vi "InitFpga.vi"(6 "bitfile path":path, 8 "error in (no error)":errorcluster, 10 "Device Name":refnum<k15>="RIO0", 11 "FPGA ref":T1) -> (0 "error out":errorcluster, 2 "session handle out":refnum<k15>, 3 "FPGA ref out":T1)   [LabVIEW 2025]
uses:
  <vilib>/rvi/interface/nirviReadWriteControl/nirviReadWriteControl.xnode
  NiFpgaLv.dll
  <vilib>/Utility/error.llb/Error Cluster From Error Code.vi
  <vilib>/rvi/interface/Simulation/niFpgaSimulationCallBeginRW.vi
  <vilib>/rvi/errors/niLvFpgaAdjustHostInterfaceError.vi
  <vilib>/rvi/interface/nirviMethod/nirviMethod.xnode
  <vilib>/rvi/errors/niLvFpgaMergeErrorWithErrorCode.vi
  x410-fpga-ref.ctl
  <vilib>/FPGAPlugInAG/Dynamic/niLvFpga_ConfigureFifo_Dynamic.vi
  <vilib>/FPGAPlugInAG/Dynamic/niLvFpga_StartFifo_Dynamic.vi
panel:
  out "Actual Depth":u32
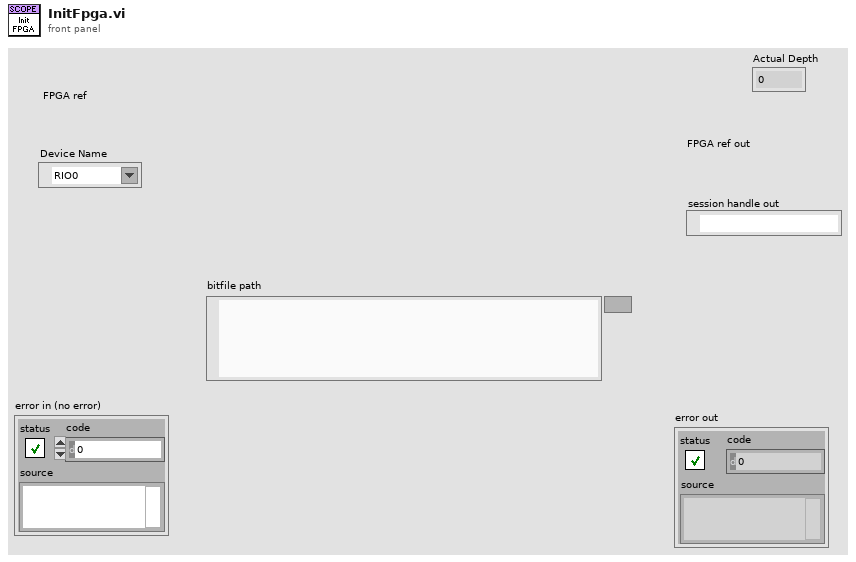
[diagram p1: front panel]
types:
  T1 = typedef "x410-fpga-ref.ctl" = refnum<k20>
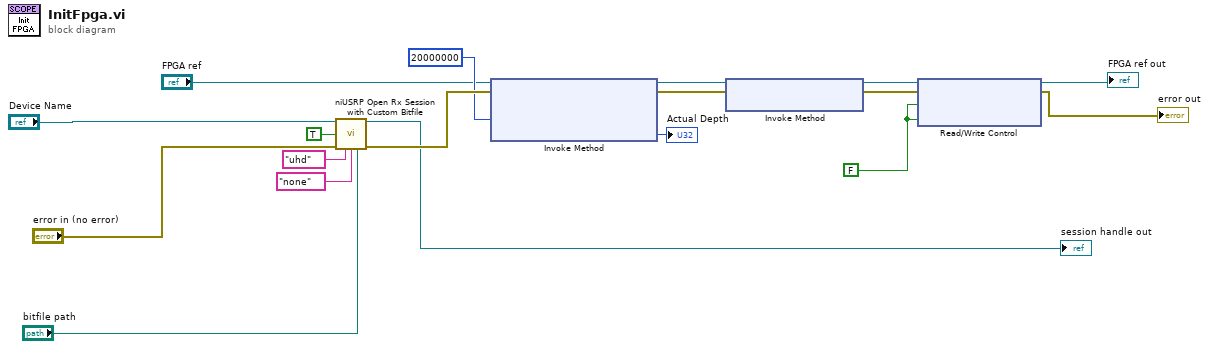
[diagram p0: block diagram]
diagram:
  w4 = FALSE ("Acquisition running")
  n1 = call <instrlib>:"niUSRP Open Rx Session with Custom Bitfile.vi"("device names"="Device Name", "reset"=TRUE, "error in (no error)"="error in (no error)", "config"="uhd", "streaming"="none", "bitfile path"="bitfile path") -> ("session handle out"=→"session handle out":refnum<k15>, "error out"=w14:errorcluster)  [unwired: 8 in]
  n2 = xnode "Invoke Method"("FPGA VI Reference In"="FPGA ref", "error in"=w14, "Requested Depth"=u32 20000000 ("Depth")) -> ("FPGA VI Reference Out"=w11:T1, "error out"=w12:errorcluster, "Actual Depth"=→"Actual Depth":u32)
  n3 = xnode "Invoke Method"("FPGA VI Reference In"=w11, "error in"=w12) -> ("FPGA VI Reference Out"=w15:T1, "error out"=w5:errorcluster)
  n4 = xnode ("Read/Write Control")("FPGA VI Reference In"=w15, "error in"=w5, "Acquisition running"=w4, "Trigger Acquisition"=w4) -> ("FPGA VI Reference Out"=→"FPGA ref out":T1, "error out"=→"error out":errorcluster)
